vi "circle-area-perimeter.vi"() -> ()   [LabVIEW 2025]
panel:
  out "Area":dbl
  out "Perimeter":dbl
  in  "r":dbl
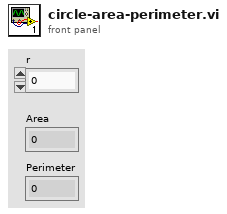
[diagram p1: front panel]
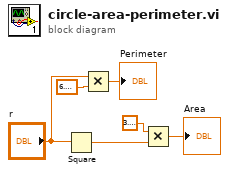
[diagram p0: block diagram]
diagram:
  n1 = Square(x="r") -> (x^2=w5:dbl)
  n2 = Multiply(x="r", y=6.283185307179586) -> (x*y=→"Perimeter":dbl)
  n3 = Multiply(x=3.141592653589793, y=w5) -> (x*y=→"Area":dbl)
